vi "Configure Digital Start Trigger.vi"(8 "error in (no error)":errorcluster, 10 "Params":variant, 11 "NI DAQmx Base in":refnum<class "NI DAQmx Base.lvclass">) -> (0 "error out":errorcluster, 3 "NI DAQmx Base out":refnum<class "NI DAQmx Base.lvclass">)   [LabVIEW 2020, in "NI DAQmx.lvlib" / "NI DAQmx Base.lvclass"]
uses:
  NI DAQmx Base.lvclass
  NI Analog Output/TypeDefs/Trigger Config.ctl
  NI Analog Output/NI Analog Output.lvclass
  <resource>/objmgr/daqmx.rc
  <vilib>/DAQmx/configure/trigger.llb/DAQmx Start Trigger (None).vi
  <vilib>/DAQmx/configure/trigger.llb/DAQmx Start Trigger (Analog Edge).vi
  <vilib>/DAQmx/configure/trigger.llb/DAQmx Start Trigger (Digital Edge).vi
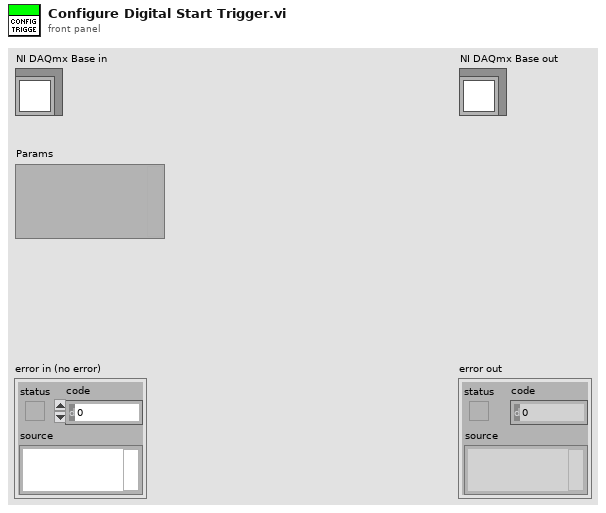
[diagram p1: front panel]
types:
  T1 = typedef "NI DAQmx.lvlib/NI Analog Output.lvclass/Trigger Config.ctl" = cluster{"trigger type":string, "source":string, "slope":i32, "analog level":dbl, "analog hysteresis":dbl}
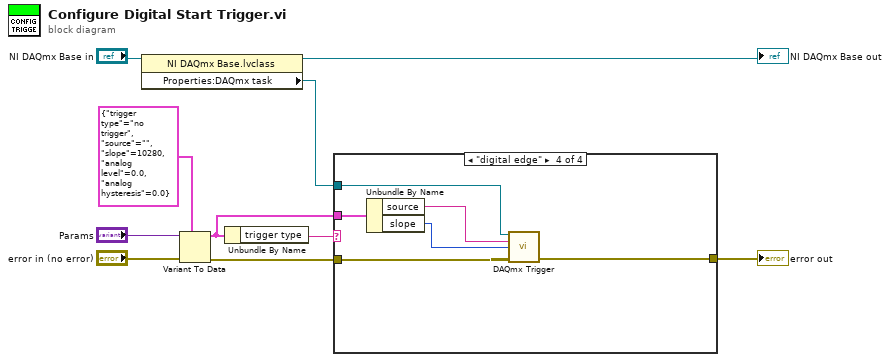
[diagram p0: block diagram]
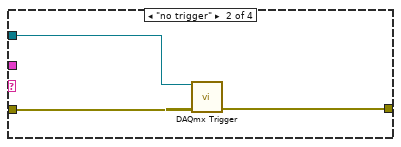
[diagram p3: hidden frame]
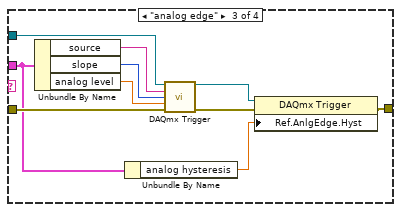
[diagram p4: hidden frame]
diagram:
  n1 = property class="NI DAQmx Base.lvclass"(reference="NI DAQmx Base in") -> (reference out=→"NI DAQmx Base out":refnum<class "NI DAQmx Base.lvclass">, "Properties:DAQmx task"=w10:refnum<k21>)  [unwired: 1 in, 1 out]
  n2 = Variant To Data(error in="error in (no error)", type=T1 {"trigger type"="no trigger", "source"="", "slope"=10280, "analog level"=0.0, "analog hysteresis"=0.0}, Variant="Params") -> (data=w6:T1, error out=w9:errorcluster)
  n3 = Unbundle By Name(w6) -> ("trigger type"=w7:string)
  n4 = case shown="\"digital edge\"" w7 {
    tunnel: [w11 w14 w17 w30] -> w1
    tunnel: w10 -> [_ w13 w23 w29]
    tunnel: w9 -> [w11 w12 w24 w28]
    tunnel: w6 -> [_ _ w16 w27]
    frame Default {
      # "invalid type"
    }
    frame "no trigger" {
      n5 = call-poly <vilib>:"DAQmx Trigger.vi"("task/channels in"=w13, "error in"=w12) -> ("error out"=w14:errorcluster)  [unwired: 12 in, 1 out]
    }
    frame "analog edge" {
      n6 = Unbundle By Name(w16) -> ("source"=w22:string, "slope"=w21:i32, "analog level"=w20:dbl)
      n7 = Unbundle By Name(w16) -> ("analog hysteresis"=w15:dbl)
      n8 = call-poly <vilib>:"DAQmx Trigger.vi"("task/channels in"=w23, "source"=w22, "slope"=w21, "level"=w20, "error in"=w24) -> ("task out"=w18:refnum<k21>, "error out"=w19:errorcluster)  [unwired: 9 in]
      n9 = property class="DAQmx Trigger"(reference=w18, error in=w19, "Ref.AnlgEdge.Hyst"=w15) -> (error out=w17:errorcluster)  [unwired: 1 out]
    }
    frame "digital edge" {
      n10 = Unbundle By Name(w27) -> ("source"=w25:string, "slope"=w26:i32)
      n11 = call-poly <vilib>:"DAQmx Trigger.vi"("task/channels in"=w29, "source"=w25, "edge"=w26, "error in"=w28) -> ("error out"=w30:errorcluster)  [unwired: 10 in, 1 out]
    }
  }
  "error out" <- w1
